vi "Populate Single Control (Variant).vi"(5 "Clust Refnum":refnum<vi>, 6 "VI Refnum":refnum<vi>, 7 "Prefix":string, 8 "error in (no error)":errorcluster, 9 "Values":variant[](array[variant]), 10 "Keys":string[](array[string]), 11 "Ctl Refnum":refnum<vi>) -> (0 "error out":errorcluster, 1 "Variant":variant, 3 "Ctl Refnum out":refnum<vi>, 4 "VI Refnum":refnum<vi>)   [LabVIEW 2017]
panel:
  in  "type specifier":refnum<vi>
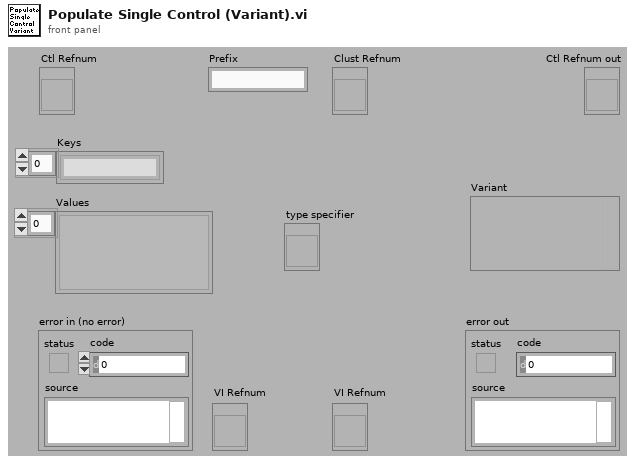
[diagram p1: front panel]
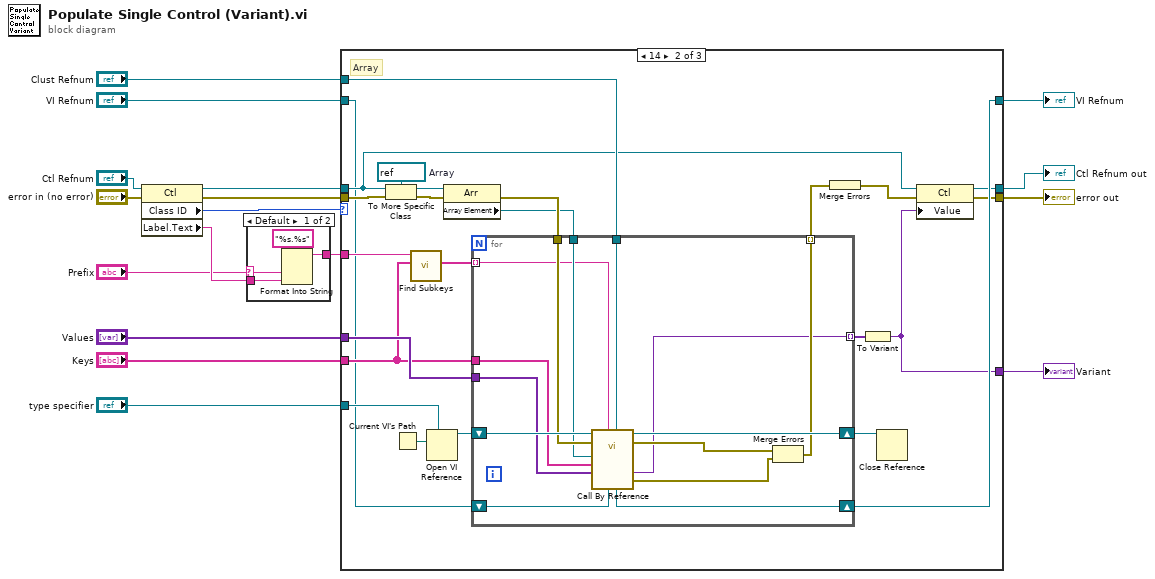
[diagram p0: block diagram]
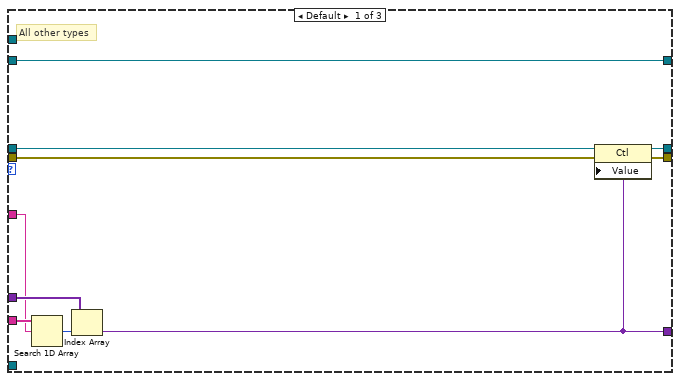
[diagram p3: hidden frame]
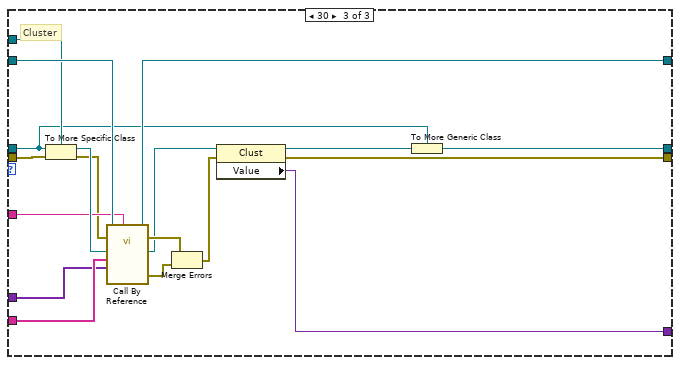
[diagram p4: hidden frame]
diagram:
  n1 = property class="Ctl"(reference="Ctl Refnum", error in="error in (no error)") -> (reference out=w9:refnum<vi>, error out=w10:errorcluster, "Class ID"=w8:u32, "Label.Text"=w6:string)
  n2 = case shown="Default" "Prefix" {
    selector: "Prefix" -> [w18 _]
    tunnel: [w21 w22] -> w17
    tunnel: w6 -> [w20 w22]
    frame Default {
      n3 = Format Into String(format string="%s.%s", w18, w20) -> (resulting string=w21:string)  [unwired: 2 in, 1 out]
    }
    frame "" {
    }
  }
  n4 = case shown="14" w8 {
    tunnel: "VI Refnum" -> [w28 w34 w87]
    tunnel: w9 -> [w25 w44 w79]
    tunnel: w10 -> [w31 w56 w88]
    tunnel: w17 -> [w24 w41 w82]
    tunnel: "Values" -> [w32 w52 w84]
    tunnel: "Keys" -> [w27 w40 w85]
    tunnel: [w28 w53 w86] -> w13
    tunnel: [w30 w43 w80] -> w16
    tunnel: [w29 w35 w71] -> w15
    tunnel: "Clust Refnum" -> [_ w54 w81]
    tunnel: [w23 w42 w74] -> w4
    tunnel: "type specifier" -> [_ w47 _]
    frame Default {
      # "All other types"
      n5 = Search 1D Array(1D array=w27, element=w24) -> (index of element=w26:i32)  [unwired: 1 in]
      n6 = Index Array(array=w32, index=w26) -> (element=w23:variant)
      n7 = property class="Ctl"(reference=w25, error in=w31, "Value"=w23) -> (reference out=w30:refnum<vi>, error out=w29:errorcluster)
    }
    frame 14 {
      w55 = refnum<vi> refnum  # Array
      # "Array"
      n8 = To More Specific Class(target class=w55, reference=w44, error in=w56) -> (specific class reference=w50:refnum<vi>, error out=w37:errorcluster)
      n9 = Current VI's Path() -> (path=w49:path)
      n10 = call "Find Subkeys.vi"("Keys"=w40, "Key Root"=w41) -> ("Subkeys"=w51:string[])  [unwired: 9 in]
      n11 = Open VI Reference(type specifier VI Refnum (for type only)=w47, vi path=w49) -> (vi reference=w48:refnum<vi>)  [unwired: 4 in, 1 out]
      n12 = property class="Arr"(reference=w50, error in=w37) -> (error out=w39:errorcluster, "Array Element"=w38:refnum<vi>)  [unwired: 1 out]
      n13 = for {
        tunnel: w40 -> [w69]
        tunnel: w52 -> [w68]
        tunnel: w54 -> [w67]
        tunnel: w38 -> [w63]
        tunnel: w39 -> [w64]
        tunnel: [w61] -> w45 mode=indexing
        tunnel: w51 -> [w60] mode=indexing
        shift-right: [w59] -> w53
        shift-left: w34 -> [w58]
        shift-right: [w66] -> w46
        shift-left: w48 -> [w70]
        tunnel: [w57] -> w33 mode=indexing
        n14 = call-by-ref "?"(reference=w70, error in=w64, "Clust Refnum"=w67, "VI Refnum"=w58, "Prefix"=w60, "Values"=w68, "Keys"=w69, "Ctl Refnum"=w63) -> (reference out=w66:refnum<vi>, error out=w62:errorcluster, 0:"error out"=w65:errorcluster, "Variant"=w57:variant, "VI Refnum"=w59:refnum<vi>)  [unwired: 2 in, 1 out]
        n15 = Merge Errors(w62, w65) -> (w61:errorcluster)
      }
      n16 = Merge Errors(w45) -> (w36:errorcluster)
      n17 = To Variant(anything=w33) -> (Variant=w42:variant)
      n18 = Close Reference(reference=w46) -> ()  [unwired: 1 in, 1 out]
      n19 = property class="Ctl"(reference=w44, error in=w36, "Value"=w42) -> (reference out=w43:refnum<vi>, error out=w35:errorcluster)
    }
    frame 30 {
      # "Cluster"
      n20 = To More Specific Class(target class=w81, reference=w79, error in=w88) -> (specific class reference=w83:refnum<vi>, error out=w72:errorcluster)
      n21 = call-by-ref "?"(reference=w87, error in=w72, "Prefix Name"=w82, "Values"=w84, "Keys"=w85, "Clust Refnum"=w83) -> (reference out=w86:refnum<vi>, error out=w77:errorcluster, 0:"error out"=w78:errorcluster, "Cluster Refnum (Dup)"=w76:refnum<vi>)  [unwired: 6 in]
      n22 = Merge Errors(w77, w78) -> (w73:errorcluster)
      n23 = property class="Clust"(reference=w76, error in=w73) -> (reference out=w75:refnum<vi>, error out=w71:errorcluster, "Value"=w74:variant)
      n24 = To More Generic Class(target class=w79, reference=w75) -> (generic class reference=w80:refnum<vi>)
    }
  }
  "Ctl Refnum out" <- w16
  "error out" <- w15
  "VI Refnum" <- w13
  "Variant" <- w4
